vi "Write CurrentState.vi"(8 "error in (no error)":errorcluster, 10 "State.lvclass":refnum<class "State.lvclass">, 11 "System in":refnum<class "System.lvclass">) -> (0 "error out":errorcluster, 3 "System out":refnum<class "System.lvclass">)   [LabVIEW 2013, in "System.lvclass"]
uses:
  System.lvclass
  States/State/State.lvclass
  Commands/Command/Command.lvclass
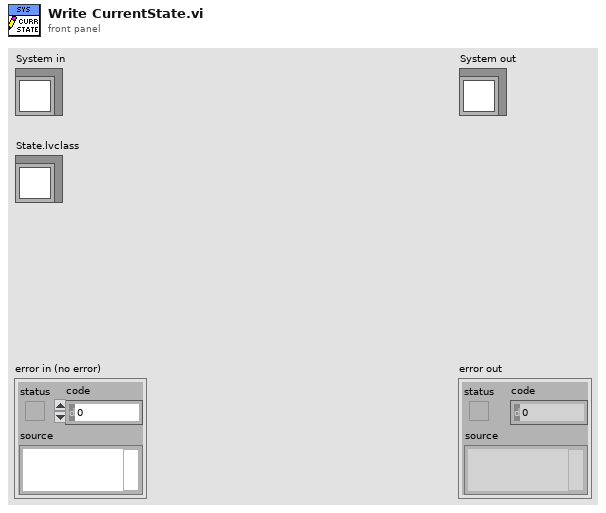
[diagram p1: front panel]
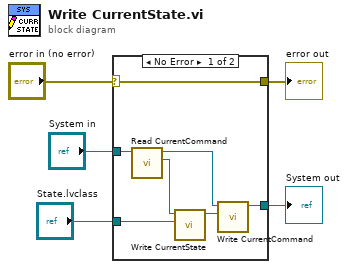
[diagram p0: block diagram]
diagram:
  n1 = case shown="No Error" "error in (no error)" {
    selector: "error in (no error)" -> [w12 w13]
    tunnel: [w12 w13] -> w4
    tunnel: [w6 w14] -> w2
    tunnel: "System in" -> [w7 w14]
    tunnel: "State.lvclass" -> [w10 _]
    frame No Error {
      n2 = call-dynamic "Read CurrentCommand.vi"("System in"=w7) -> ("Command.lvclass"=w11:refnum<class "Command.lvclass">, "System out"=w8:refnum<class "System.lvclass">)  [unwired: 8 in, 1 out]
      n3 = call-dynamic "Write CurrentState.vi"("State.lvclass"=w10, "Command in"=w11) -> ("Command out"=w9:refnum<class "Command.lvclass">)  [unwired: 8 in, 1 out]
      n4 = call-dynamic "Write CurrentCommand.vi"("Command.lvclass"=w9, "System in"=w8) -> ("System out"=w6:refnum<class "System.lvclass">)  [unwired: 8 in, 1 out]
    }
    frame Error {
    }
  }
  "error out" <- w4
  "System out" <- w2
